vi "UHR-Fleezers Control (host) - 10.7.vi"() -> ()   [LabVIEW 2011] (continued)
        n1732 = Equal?(x=w2649, y=0) -> (x = y?=w2647:bool)
      }
      n1733 = local write "Stop All"(FALSE ("Stop All")) -> ()
    }
    frame #1 {
      n1734 = call "DMR_Init.vi"() -> ()  [unwired: 3 out]
    }
    frame #2 {
      # "Setting the destination format to Mono8 makes sure that the image can be displayed in the intensity plot."
      n1735 = call "DMR_GetDevice.vi"("search string IN"="DE019116701") -> ("device handle OUT"=w2672:i32)  [unwired: 4 in, 2 out]
      n1736 = call "DMR_OpenDevice.vi"("device handle IN"=w2672) -> ("driver handle OUT"=w2655:i32)  [unwired: 4 out]
      n1737 = call "DMR_FindList.vi"("flags IN"=u32 0 ("flags"), "list name IN"="" ("String"), "list type IN"=T31."camera descriptions", "driver handle IN"=w2655) -> ("list handle OUT"=w2658:i32)  [unwired: 2 out]
      n1738 = call "DMR_FindList.vi"("flags IN"=u32 0 ("flags"), "list name IN"="Base", "list type IN"=T31."setting", "driver handle IN"=w2655) -> ("list handle OUT"=w2656:i32)  [unwired: 2 out]
      n1739 = call "OBJ_GetHandle.vi"("object name IN"="VideoStandard", "list handle IN"=w2658) -> ("object handle OUT"=w2652:i32)  [unwired: 3 out]
      n1740 = call "OBJ_GetHandle.vi"("object name IN"="PixelFormat", "list handle IN"=w2656) -> ("object handle OUT"=w2666:i32)  [unwired: 3 out]
      n1741 = call "OBJ_SetS.vi"("value index IN"=0, "value IN"="NTSC M", "object handle IN"=w2652) -> ()  [unwired: 2 out]
      n1742 = call "OBJ_SetS.vi"("value index IN"=0, "value IN"="Mono8" ("value"), "object handle IN"=w2666) -> ()  [unwired: 2 out]
      n1743 = call "OBJ_GetHandle.vi"("object name IN"="VideoChannel", "list handle IN"=w2656) -> ("object handle OUT"=w2662:i32)  [unwired: 3 out]
      n1744 = while {
        tunnel: [w2677] -> w2654
        tunnel: w2655 -> [w2674]
        stop <- w2675 continue-if-true
        n1745 = call "DMR_ImageRequestSingle.vi"("request control IN"=0, "driver handle IN"=w2674) -> ("error code OUT"=w2676:i32, "driver handle OUT"=w2677:i32)  [unwired: 2 out]
        n1746 = Equal To 0?(x=w2676) -> (x = 0?=w2675:bool)
      }
      n1747 = call "OBJ_SetI.vi"("value index IN"=0, "value IN"=3 ("Video channel"), "object handle IN"=w2662) -> ()  [unwired: 2 out]
    }
    frame #3 {
      w2683 = T17 0 items=["Grayscale (U8)", "Grayscale (I16)", "Grayscale (SGL)", "Complex (CSG)", "RGB (U32)", "HSL (U32)", "RGB (U64)"] ("Image Type")
      w2691 = T17 0 items=["Grayscale (U8)", "Grayscale (I16)", "Grayscale (SGL)", "Complex (CSG)", "RGB (U32)", "HSL (U32)", "RGB (U64)"] ("Image Type")
      n1748 = for "Create Greyscale map" {
        N: 256 -> [_]
        tunnel: [w2697] -> w2680 mode=indexing
        workers-P: _ -> [_]
        i -> [w2700]
        n1749 = To Unsigned Byte Integer(number=w2700) -> (unsigned 8bit integer=w2696:u8)
        n1750 = Join Numbers(hi=w2696, lo=w2696) -> ((hi.lo)=w2699:u16)
        n1751 = Join Numbers(hi=w2696, lo=w2696) -> ((hi.lo)=w2698:u16)
        n1752 = Join Numbers(hi=w2699, lo=w2698) -> ((hi.lo)=w2697:u32)
      }
      n1753 = call "IMAQ Create"("Image Name"="Scaled video", "Image Type"=w2683) -> ("New Image"=w2682:T2)  [unwired: 2 in, 2 out]
      n1754 = call "IMAQ Create"("Image Name"="Main video", "Image Type"=w2691) -> ("New Image"=w2692:T2)  [unwired: 2 in, 2 out]
      n1755 = node-c288(0 ("Processor")) -> (w2690:T21)  [unwired: 3 out]
      n1756 = Initialize Array(u32 0 ("Window Number (0...15)"), 480 ("dimension size"), 640 ("dimension size")) -> (w2685:u32[][])
      n1757 = timed-loop {
        tunnel: w2695 -> [w2717]
        tunnel: [w2716] -> w2694
        tunnel: w2692 -> [w2715]
        timing: w2690 -> [_]
        timing-out: [_] -> w2689
        tunnel: w2685 -> [w2704]
        tunnel: w2682 -> [w2702]
        tunnel: w2680 -> [w2701]
        stop <- w2703 stop-if-true
        # "This block performs the \nactual image capture."
        n1758 = node-c288() -> ()  [unwired: 2 out]
        n1759 = local read "Stop All"() -> (w2703:bool)
        n1760 = Reciprocal(x="Video Capture Rate (Hz)") -> (1/x=w2707:dbl)
        n1761 = Multiply(x=w2707, y=1000.0) -> (x*y=w2705:dbl)
        n1762 = call "DMR_ImageRequestWaitFor.vi"("queue number IN"=0, "timeout(ms) IN"=500, "driver handle IN"=w2717) -> ("error code OUT"=w2721:i32, "request number OUT"=w2718:i32, "driver handle OUT"=w2719:i32)
        n1763 = feedback #1(T32 refnum ("Avi Refnum")) -> (w2709:T32)
        n1764 = case shown="True" "New Video File" {
          tunnel: [T32 refnum ("Avi Refnum") w2738] -> w2711
          tunnel: [FALSE TRUE] -> w2712
          tunnel: w2709 -> [_ w2734]
          frame False {
          }
          frame True {
            n1765 = call "Create new save file.vi"("Ext"=".avi" ("string"), "Index In"="Video Index") -> ("Path Out"=w2730:path, "Index Out"=w2731:dbl)  [unwired: 1 in]
            "Path Out" <- w2730
            n1766 = Not Equal?(x=w2734, y=T32 refnum ("Avi Refnum")) -> (x != y?=w2735:bool)
            n1767 = Increment(x=w2731) -> (x+1=w2740:dbl)
            n1768 = case shown="True" w2735 {
              tunnel: w2734 -> [_ w2741]
              frame False {
              }
              frame True {
                n1769 = call "IMAQ AVI Close"("Avi Refnum"=w2741) -> ()  [unwired: 1 in, 10 out]
              }
            }
            n1770 = local write "Video Index"(w2740) -> ()
            n1771 = call "IMAQ AVI Create"("Frames Per Second"=u32 30, "AVI Path"=w2730) -> ("Avi Refnum"=w2738:T32)  [unwired: 5 in, 4 out]
          }
        }
        n1772 = Equal To 0?(x=w2721) -> (x = 0?=w2720:bool)
        n1773 = Select(t=w2711, s=w2712, f=w2709) -> (s? t:f=w2710:T32)
        n1774 = feedback-in #1(w2710) -> ()
        n1775 = case shown="True" w2720 {
          tunnel: w2719 -> [w2742 w2767]
          tunnel: w2718 -> [_ w2766]
          tunnel: [w2742 w2763] -> w2716
          tunnel: w2715 -> [_ w2747]
          tunnel: w2704 -> [_ w2751]
          tunnel: w2710 -> [_ w2749]
          tunnel: w2702 -> [_ w2744]
          tunnel: w2701 -> [_ w2743]
          frame False {
          }
          frame True {
            w2757 = u32 0 ("X-offset IN")
            n1776 = call "DMR_GetImageRequestBufferData.vi"("driver handle IN"=w2767, "request number IN"=w2766) -> ("width OUT"=w2756:i32, "height OUT"=w2755:i32, "driver handle OUT"=w2762:i32, "request number OUT"=w2761:i32, "bytes per pixel OUT"=w2758:i32)  [unwired: 13 out]
            n1777 = call "DMR_GetImageRequestBufferImageData.vi"("driver handle IN"=w2762, "request number IN"=w2761, "bytes per pixel IN"=w2758, "X-offset IN"=w2757, "Y-offset IN"=w2757, "height IN"=w2755, "width IN"=w2756) -> ("driver handle OUT"=w2760:u32, "request number OUT"=w2759:u32, "image OUT"=w2752:u32[][])  [unwired: 10 out]
            n1778 = call "DMR_ImageRequestUnlock.vi"("request number IN"=w2759, "driver handle IN"=w2760) -> ("driver handle OUT"=w2765:i32)  [unwired: 1 in, 2 out]
            n1779 = case shown="True" "Averaging" {
              tunnel: w2752 -> [w2803 w2808]
              tunnel: [w2803 w2807] -> w2748
              tunnel: w2751 -> [_ w2805]
              frame False {
              }
              frame True {
                (unwired) 1
                w2813 = 1
                n1780 = feedback #2(w2805) -> (w2804:u32[][])
                n1781 = Add(x=w2808, y=w2804) -> (x+y=w2809:u32[][])
                n1782 = Select(t=w2805, s="Reset Averaging", f=w2809) -> (s? t:f=w2811:u32[][])
                n1783 = feedback-in #2(w2811) -> ()
                n1784 = feedback #3(w2813) -> (w2806:i32)
                n1785 = Divide(x=w2809, y=w2806) -> (x/y=w2810:dbl[][])
                n1786 = Increment(x=w2806) -> (x+1=w2814:i32)
                n1787 = To Unsigned Long Integer(number=w2810) -> (unsigned 32bit integer=w2807:u32[][])
                n1788 = Select(t=w2813, s="Reset Averaging", f=w2814) -> (s? t:f=w2812:i32)
                n1789 = feedback-in #3(w2812) -> ()
              }
            }
            n1790 = call "DMR_ImageRequestSingle.vi"("request control IN"=0, "driver handle IN"=w2765) -> ("driver handle OUT"=w2763:i32)  [unwired: 3 out]
            n1791 = disable-structure shown="Disabled" {
              disable-tunnel: w2748 -> [w2780 _]
              disable-tunnel: w2744 -> [w2779 _]
              frame Disabled {
                n1792 = To Double Precision Float(number=w2780) -> (double precision float=w2778:dbl[][])
                n1793 = In Range and Coerce(upper limit="Intensity Upper", x=w2778, lower limit="Intensity Lower") -> (coerced(x)=w2777:dbl[][])  [unwired: 1 out]
                n1794 = Subtract(x="Intensity Upper", y="Intensity Lower") -> (x-y=w2774:dbl)
                n1795 = Subtract(x=w2777, y="Intensity Lower") -> (x-y=w2775:dbl[][])
                n1796 = Divide(x=w2775, y=w2774) -> (x/y=w2776:dbl[][])
                n1797 = Multiply(x=255.0, y=w2776) -> (x*y=w2772:dbl[][])
                n1798 = To Unsigned Byte Integer(number=w2772) -> (unsigned 8bit integer=w2781:u8[][])
                n1799 = call "IMAQ ArrayToImage"("Image Pixels (U8)"=w2781, "Image"=w2779) -> ("Image Out"=w2768:T2)  [unwired: 4 in, 5 out]
                n1800 = First Call?() -> (First Call?: T/F=w2769:bool)
                n1801 = case shown="True" w2769 {
                  tunnel: w2768 -> [w2782 w2793]
                  frame False {
                    n1802 = flat-sequence {
                      tunnel: w2782 -> [w2788]
                      frame #0 {
                        w2785 = FALSE ("Get/Set Status? (Set)")
                        w2784 = 0 ("Window Number (0...15)")
                        n1803 = call "IMAQ WindSize"("Get/Set Status? (Set)"=w2785, "Window Number"=w2784) -> ("Width & Height out"=→"Window Size":cluster{"Width":i32, "Height":i32})  [unwired: 4 in, 2 out]
                        n1804 = call "IMAQ WindMove"("Window Number (0...15)"=w2784, "Get/Set Status? (Set)"=w2785) -> ("Coordinates (screen)"=→"Window Position":cluster{"X Position":i32, "Y Position":i32})  [unwired: 3 in, 1 out]
                        n1805 = call "IMAQ WindDraw"("Resize to Image Size? (Y)"=FALSE, "Window Number (0...15)"=w2784, "Image"=w2788) -> ()  [unwired: 7 in, 2 out]
                      }
                      frame #1 {
                        n1806 = call "IMAQ WindZoom 2"("Center Point"="Center Point", "Zoom to Fit? (False)"=FALSE, "Zoom Factor"="Zoom Factor") -> ()  [unwired: 5 in, 4 out]
                      }
                    }
                  }
                  frame True {
                    n1807 = flat-sequence {
                      tunnel: w2793 -> [w2796]
                      tunnel: [w2794] -> w2792
                      tunnel: w2792 -> [w2798]
                      frame #0 {
                        w2795 = TRUE ("Resize to Image Size? (Y)")
                        w2794 = 0 ("Window Number (0...15)")
                        n1808 = call "IMAQ WindNonTearing"("Window Number"=w2794, "NonTearing? (True)"=w2795) -> ()  [unwired: 8 in, 2 out]
                        n1809 = call "IMAQ WindDraw"("Resize to Image Size? (Y)"=w2795, "Window Number (0...15)"=w2794, "Image"=w2796) -> ()  [unwired: 7 in, 2 out]
                      }
                      frame #1 {
                        n1810 = call "IMAQ WindSize"("Scrollbars? (N)"=FALSE, "Width & Height"="Initial Window Size", "Window Number"=w2798) -> ()  [unwired: 3 in, 3 out]
                        n1811 = call "IMAQ WindMove"("Window Number (0...15)"=w2798, "Coordinates (screen)"="Initial Window Position") -> ()  [unwired: 3 in, 2 out]
                      }
                    }
                  }
                }
              }
              frame Enabled {
              }
            }
            n1812 = To Unsigned Byte Integer(number=w2748) -> (unsigned 8bit integer=w2746:u8[][])
            n1813 = call "IMAQ ArrayToImage"("Image Pixels (U8)"=w2746, "Image"=w2747) -> ("Image Out"=w2745:T2)  [unwired: 4 in, 5 out]
            "Primary Video Display" <- w2745
            n1814 = case shown="True" "Save Video" {
              tunnel: w2749 -> [_ w2802]
              tunnel: w2745 -> [_ w2801]
              frame False {
              }
              frame True {
                n1815 = call "IMAQ AVI Write Frame"("Image"=w2801, "Avi Refnum"=w2802) -> ()  [unwired: 2 in, 8 out]
              }
            }
            n1816 = case shown="True" "Save Image" {
              tunnel: w2746 -> [_ w2817]
              tunnel: w2743 -> [_ w2816]
              frame False {
              }
              frame True {
                n1817 = call <vilib>:"Flatten Pixmap.vi"("colors"=w2816, "8-bit pixmap"=w2817) -> ("image data"=w2823:T33)  [unwired: 4 in, 5 out]
                n1818 = call "Create new save file.vi"("Insert"="video_frame_" ("string"), "Ext"=".bmp" ("string"), "Index In"="Image Index") -> ("Path Out"=w2819:path, "Index Out"=w2824:dbl)
                n1819 = Increment(x=w2824) -> (x+1=w2818:dbl)
                n1820 = local write "Image Index"(w2818) -> ()
                n1821 = call <vilib>:"Write BMP File.vi"("image data"=w2823, "path to BMP file"=w2819) -> ()  [unwired: 1 in, 9 out]
              }
            }
          }
        }
        n1822 = node-c288(w2705) -> ()  [unwired: 1 out]
      }
      n1823 = node-c288(w2689) -> ()  [unwired: 1 out]
      n1824 = call "DMR_CloseDevice.vi"("driver handle IN"=w2694) -> ()  [unwired: 1 in, 4 out]
    }
    frame #4 {
      n1825 = call "DMR_Close.vi"() -> ()  [unwired: 1 out]
    }
  }
  n1826 = node-c288(i64 1 ("Period"), 1 ("Processor")) -> (w175:T21)  [unwired: 2 out]
  n1827 = timed-loop "Acquire Data" {
    tunnel: w50 -> [w3123]
    tunnel: w49 -> [w3122]
    tunnel: [w3152] -> w270
    tunnel: [w3147] -> w268
    timing: w175 -> [_]
    timing-out: [_] -> w174
    tunnel: w69 -> [w2960]
    stop <- "Stop All" stop-if-true
    w2875 = "Initialize"
    w2945 = "NI_ChannelName" ("name")
    n1828 = node-c288() -> ()  [unwired: 2 out]
    n1829 = First Call?() -> (First Call?: T/F=w2910:bool)
    n1830 = Or(x="Reset", y=w2910) -> (x .or. y?=w2911:bool)
    n1831 = local read "Flushing P1"() -> (w2829:bool)
    n1832 = case "Reset data stream" shown="True" w2911 {
      tunnel: w3123 -> [w4128 w4136]
      tunnel: w3122 -> [w4127 w4135]
      tunnel: [w4128 w4130] -> w3118
      tunnel: [w4127 w4129] -> w3117
      frame False {
      }
      frame True {
        w4133 = TRUE ("AI to FIFO")
        n1833 = local write "Overflow (data lost)"(FALSE ("Overflow (data lost)")) -> ()
        n1834 = call "reset FPGA DMA.vi"("error in"=w4135, "FPGA VI Reference In"=w4136) -> ("error out"=w4131:errorcluster, "FPGA VI Reference Out"=w4132:T19)
        n1835 = xnode "Read/Write Control"("FPGA VI Reference In"=w4132, "error in"=w4131, "AI to FIFO"=w4133, "APD to FIFO"=w4133) -> ("FPGA VI Reference Out"=w4130:T19, "error out"=w4129:errorcluster)
      }
    }
    n1836 = case shown="True" w2829 {
      frame False {
      }
      frame True {
        n1837 = local read "Flush rate (uL/m) P1"() -> (w3169:dbl)
        n1838 = local read "HP1 Flush Time (s)"() -> (w3178:dbl)
        n1839 = local read "DMA Update Period (s)"() -> (w3172:dbl)
        n1840 = Divide(x=w3169, y=60.0) -> (x/y=w3170:dbl)
        n1841 = Divide(x=w3178, y=w3172) -> (x/y=w3167:dbl)
        n1842 = feedback #4(0) -> (w3176:i32)
        n1843 = Increment(x=w3176) -> (x+1=w3166:i32)
        n1844 = Greater?(x=w3166, y=w3167) -> (0:w3175:bool)
        n1845 = Compound Arithmetic op=MULTIPLY(w3172, w3166, w3170) -> (→"P1 Flush Volume (uL)":dbl)
        n1846 = Divide(x=w3166, y=w3167) -> (x/y=→"P1 Flushing Bar":dbl)
        n1847 = case shown="True" w3175 {
          tunnel: w3166 -> [w3179 _]
          tunnel: [w3179 0] -> w3174
          frame False {
          }
          frame True {
            w3180 = FALSE ("Flushing P1")
            n1848 = local write "Inject Pump 1"(w3180) -> ()
            n1849 = local write "Flushing P1"(w3180) -> ()
            n1850 = property on="Clear Volume P1" class="Bool (strict)"("Val(Sgnl)"=TRUE ("Value (Signaling)")) -> ()  [unwired: 2 in, 2 out]
          }
        }
        n1851 = feedback-in #4(w3174) -> ()
      }
    }
    n1852 = Or(x="Start AOD Scan", y="Trap Raster Scan") -> (x .or. y?=w3068:bool)
    n1853 = case "Start AOM raster scan" shown="True" w3068 {
      tunnel: w3118 -> [w3978 w3988]
      tunnel: w3117 -> [w3977 w3987]
      tunnel: [w3978 w3981] -> w3116
      tunnel: [w3977 w3980] -> w3115
      frame False {
      }
      frame True {
        n1854 = case shown="True" "Restart DMA? (AOD)" {
          tunnel: [w4026 w4028] -> w3982
          tunnel: [w4025 w4027] -> w3983
          tunnel: w3988 -> [w4026 w4030]
          tunnel: w3987 -> [w4025 w4029]
          frame False {
          }
          frame True {
            n1855 = local write "Overflow (data lost)"(FALSE ("Overflow (data lost)")) -> ()
            n1856 = call "reset FPGA DMA.vi"("error in"=w4029, "FPGA VI Reference In"=w4030) -> ("error out"=w4027:errorcluster, "FPGA VI Reference Out"=w4028:T19)
          }
        }
        n1857 = local write "Trap Raster Scan"(FALSE ("Trap Raster Scan")) -> ()
        n1858 = case shown="True" "Move MCL Also?" {
          tunnel: w3983 -> [w3991 w4020]
          tunnel: w3982 -> [w3992 w4021]
          tunnel: [w3990 w4024] -> w3981
          tunnel: [w3989 w4023] -> w3980
          frame False {
            w3993 = TRUE ("AI to FIFO")
            n1859 = xnode "Read/Write Control"("FPGA VI Reference In"=w3992, "error in"=w3991, "AI to FIFO"=w3993, "APD to FIFO"=w3993, "Start scan"=w3993) -> ("FPGA VI Reference Out"=w3990:T19, "error out"=w3989:errorcluster)
          }
          frame True {
            w4017 = FALSE ("1D or 2D Scan?")
            w4022 = TRUE ("AI to FIFO")
            # "Count for MCL loop"
            # "N total cycles"
            # "N steps"
            # "V_int"
            n1860 = local read "Scan Range (nm)"() -> (w3999:dbl)
            n1861 = local read "Number of F/B Scans (AOD)"() -> (w4016:u16)
            n1862 = Sign(1:w3999) -> (0:w3998:dbl)
            n1863 = Compound Arithmetic op=MULTIPLY(w3999, "MCL Step Position Ratio", "MCL/AOM Scale Tweak") -> (w4003:dbl)
            n1864 = Negate(x=w3998) -> (-x=w3995:dbl)
            n1865 = Multiply(x=w3995, y="MCL Step Increment (V_int)") -> (x*y=w3997:dbl)
            n1866 = Divide(x=w4003, y="MCL X Cal (nm/V)") -> (x/y=w4009:dbl)
            n1867 = Multiply(x=32767.0 ("y"), y=w4009) -> (x*y=w4015:dbl)
            n1868 = local read "Total Counts (ticks)"() -> (w4000:u32)
            n1869 = local read "Cycles/step (AOD)"() -> (w4011:u64)
            n1870 = local read "Scan steps (AOD)"() -> (w4012:u64)
            n1871 = Divide(x=w4015, y=10.0) -> (x/y=w4008:dbl)
            n1872 = Divide(x=w4008, y="MCL Step Increment (V_int)") -> (x/y=w4006:dbl)
            n1873 = Absolute Value(x=w4006) -> (abs(x)=w3994:dbl)
            n1874 = Compound Arithmetic op=MULTIPLY(w4012, w4011, w4000) -> (w4007:u64)
            n1875 = local write "wait to reset values"(w4022) -> ()
            n1876 = local write "MCL Scanning"(w4022) -> ()
            n1877 = Divide(x=w4007, y=w3994) -> (x/y=w4004:dbl)
            "MCL Count" <- w4004
            n1878 = xnode "Read/Write Control"("FPGA VI Reference In"=w4021, "error in"=w4020, "Scan steps (MCL)"=w3994, "Number of scans (MCL)"=w4016, "Cycles per step (MCL)"=u64 1, "Scan freq.  increment (MCL)"=w3997, "1D or 2D Scan?"=w4017, "MCL Scan Axis"=w4017, "Cont. Scan (MCL)"=w4017, "MCL count"=w4004) -> ("FPGA VI Reference Out"=w4019:T19, "error out"=w4018:errorcluster)
            n1879 = xnode "Read/Write Control"("FPGA VI Reference In"=w4019, "error in"=w4018, "AI to FIFO"=w4022, "APD to FIFO"=w4022, "Start scan"=w4022, "Start scan (MCL)"=w4022) -> ("FPGA VI Reference Out"=w4024:T19, "error out"=w4023:errorcluster)
          }
        }
        "Raster Scanning..." <- TRUE ("Scanning...")
      }
    }
    n1880 = local read "Flushing P3"() -> (w2830:bool)
    n1881 = case "Keep track of when Harvard Pump 3 is done flushing" shown="True" w2830 {
      frame False {
      }
      frame True {
        n1882 = local read "Flush rate (uL/m) P3"() -> (w3186:dbl)
        n1883 = local read "DMA Update Period (s)"() -> (w3188:dbl)
        n1884 = local read "HP3 Flush Time (s)"() -> (w3195:dbl)
        n1885 = Divide(x=w3186, y=60.0) -> (x/y=w3184:dbl)
        n1886 = feedback #5(0) -> (w3193:i32)
        n1887 = Increment(x=w3193) -> (x+1=w3187:i32)
        n1888 = Divide(x=w3195, y=w3188) -> (x/y=w3189:dbl)
        n1889 = Greater?(x=w3187, y=w3189) -> (0:w3192:bool)
        n1890 = Compound Arithmetic op=MULTIPLY(w3188, w3187, w3184) -> (→"P3 Flush Volume (uL)":dbl)
        n1891 = case shown="True" w3192 {
          tunnel: w3187 -> [w3196 _]
          tunnel: [w3196 0] -> w3191
          frame False {
          }
          frame True {
            w3197 = FALSE ("Flushing P3")
            n1892 = local write "Inject Pump 3"(w3197) -> ()
            n1893 = local write "Flushing P3"(w3197) -> ()
            n1894 = property on="Clear Volume P3" class="Bool (strict)"("Val(Sgnl)"=TRUE ("Value (Signaling)")) -> ()  [unwired: 2 in, 2 out]
          }
        }
        n1895 = feedback-in #5(w3191) -> ()
        n1896 = Divide(x=w3187, y=w3189) -> (x/y=→"P3 Flushing Bar":dbl)
      }
    }
    n1897 = And(x="Save scans", y=w3068) -> (x .and. y?=w3114:bool)
    n1898 = Compound Arithmetic op=OR("Start MCL Scan", "Confocal Image", "Confocal Linescan") -> (w3066:bool)
    n1899 = And(x="Save Data (MCL)", y=w3066) -> (x .and. y?=w3113:bool)
    n1900 = case "Start MCL raster scan" shown="True" w3066 {
      tunnel: w3116 -> [w3595 w3611]
      tunnel: w3115 -> [w3594 w3610]
      tunnel: [w3595 w3606] -> w2958
      tunnel: [w3594 w3605] -> w2957
      tunnel: [FALSE w3604] -> w3099
      tunnel: "Start MCL Scan" -> [_ w3599]
      tunnel: "Confocal Image" -> [_ w3598]
      tunnel: "Confocal Linescan" -> [_ _]
      frame False {
      }
      frame True {
        w3604 = TRUE
        n1901 = case shown="True" "Restart DMA? (MCL)" {
          tunnel: [w3656 w3658] -> w3609
          tunnel: [w3655 w3657] -> w3608
          tunnel: w3611 -> [w3656 w3661]
          tunnel: w3610 -> [w3655 w3660]
          frame False {
          }
          frame True {
            n1902 = call "reset FPGA DMA.vi"("error in"=w3660, "FPGA VI Reference In"=w3661) -> ("error out"=w3657:errorcluster, "FPGA VI Reference Out"=w3658:T19)
            n1903 = local write "Overflow (data lost)"(FALSE ("Overflow (data lost)")) -> ()
          }
        }
        n1904 = case shown="False" w3599 {
          selector: w3599 -> [_ w3615]
          tunnel: w3598 -> [w3614 _]
          tunnel: [w3614 w3615] -> w3597
          frame False {
            n1905 = property on="2D or 1D Scan" class="Bool (strict)"("Val(Sgnl)"=w3614) -> ()  [unwired: 2 in, 2 out]
            n1906 = property on="Confocal Image" class="Bool (strict)"("Value"=FALSE ("Start Confocal Map")) -> ()  [unwired: 2 in, 2 out]
          }
          frame True {
          }
        }
        n1907 = local write "MCL Scanning"(w3604) -> ()
        n1908 = local read "AO1"() -> (w3601:dbl)
        n1909 = local read "AO2"() -> (w3600:dbl)
        n1910 = case shown="True" "Center Scan" {
          tunnel: w3609 -> [w3622 w3654]
          tunnel: w3608 -> [w3621 w3653]
          tunnel: [w3620 w3652] -> w3606
          tunnel: [w3619 w3651] -> w3605
          tunnel: [w3617 w3638] -> w3603
          tunnel: [w3616 w3637] -> w3602
          tunnel: w3601 -> [w3617 w3643]
          tunnel: w3600 -> [w3616 w3646]
          tunnel: w3597 -> [_ _]
          frame False {
            w3618 = TRUE ("AI to FIFO")
            n1911 = xnode "Read/Write Control"("FPGA VI Reference In"=w3622, "error in"=w3621, "AI to FIFO"=w3618, "APD to FIFO"=w3618, "Start scan (MCL)"=w3618) -> ("FPGA VI Reference Out"=w3620:T19, "error out"=w3619:errorcluster)
          }
          frame True {
            w3650 = TRUE ("AI to FIFO")
            n1912 = local read "Scan steps (MCL)"() -> (w3629:u64)
            n1913 = local read "Scan lines (y)"() -> (w3625:u64)
            n1914 = local read "Fast Scan Dir"() -> (w3636:bool)
            n1915 = local read "Actual MCL Inc (V)"() -> (w3626:dbl)
            n1916 = Decrement(x=w3625) -> (x-1=w3624:u64)
            n1917 = Decrement(x=w3629) -> (x-1=w3628:u64)
            n1918 = Multiply(x=w3626, y=w3624) -> (x*y=w3623:dbl)
            n1919 = Divide(x=w3623, y=2.0) -> (x/y=w3633:dbl)
            n1920 = Multiply(x=w3626, y=w3628) -> (x*y=w3627:dbl)
            n1921 = Divide(x=w3627, y=2.0) -> (x/y=w3632:dbl)
            n1922 = Select(t=w3632, s=w3636, f=w3633) -> (s? t:f=w3631:dbl)
            n1923 = Select(t=w3633, s=w3636, f=w3632) -> (s? t:f=w3635:dbl)
            n1924 = Subtract(x=w3643, y=w3635) -> (x-y=w3634:dbl)
            n1925 = Subtract(x=w3646, y=w3631) -> (x-y=w3630:dbl)
            n1926 = local read "2D or 1D Scan"() -> (w3648:bool)
            n1927 = Not(x=w3636) -> (.not. x?=w3642:bool)
            n1928 = Not(x=w3648) -> (.not. x?=w3644:bool)
            n1929 = And(x=w3636, y=w3644) -> (x .and. y?=w3645:bool)
            n1930 = And(x=w3644, y=w3642) -> (x .and. y?=w3647:bool)
            n1931 = Select(t=w3646, s=w3647, f=w3630) -> (s? t:f=w3637:dbl)
            n1932 = Select(t=w3643, s=w3645, f=w3634) -> (s? t:f=w3638:dbl)
            n1933 = call "Volt to I16.vi"("Voltage In"=w3638) -> ("I16 Voltage Out"=w3641:i16)
            n1934 = call "Volt to I16.vi"("Voltage In"=w3637) -> ("I16 Voltage Out"=w3640:i16)
            n1935 = xnode "Read/Write Control"("FPGA VI Reference In"=w3654, "error in"=w3653, "AI to FIFO"=w3650, "APD to FIFO"=w3650, "Start scan (MCL)"=w3650, "AO1"=w3641, "AO2"=w3640) -> ("FPGA VI Reference Out"=w3652:T19, "error out"=w3651:errorcluster)
          }
        }
        "Initial Y" <- w3603
        "Initial X" <- w3602
        n1936 = local write "Tab Control 6"(T3."Imaging" ("Tab Control 6")) -> ()
        "wait to reset values" <- w3604
      }
    }
    n1937 = local read "Trap Pos Elements/DMA read"() -> (w2954:u32)
    n1938 = local read "Trap AI Elements/DMA read"() -> (w3029:u32)
    n1939 = local read "APD Elements/DMA read"() -> (w2995:u32)
    n1940 = xnode "Get APD Data"("FPGA VI Reference In"=w2958, "error in"=w2957, "Number of Elements"=w2995, "Timeout (ms)"=-1) -> ("Data"=w2994:u32[], "Elements Remaining"=→"APD FIFO Elements Remaining":u32)  [unwired: 2 out]
    n1941 = xnode "Invoke Method"("FPGA VI Reference In"=w2958, "error in"=w2957, "Number of Elements"=w2954, "Timeout (ms)"=-1) -> ("Data"=w2917:u16[], "Elements Remaining"=→"Trap Pos FIFO El Remaining":u32)  [unwired: 2 out]
    n1942 = xnode "Get Trap Data"("FPGA VI Reference In"=w2958, "error in"=w2957, "Number of Elements"=w3029, "Timeout (ms)"=-1 ("Timeout")) -> ("FPGA VI Reference Out"=w2851:T19, "error out"=w2850:errorcluster, "Data"=w2918:i16[], "Elements Remaining"=w3160:u32)
    "FIFO El. Rem." <- w3160
    n1943 = local read "Trap AI FIFO Depth"() -> (w3162:u32)
    n1944 = Subtract(x=w3162, y=w3029) -> (x-y=w3161:u32)
    n1945 = Decimate 1D Array(w2917) -> (w2914:u16[], w2916:u16[], w2915:u16[])
    n1946 = Divide(x=w3160, y=w3161) -> (x/y=w3159:dbl)
    "Buffer Status" <- w3159
    n1947 = To Unsigned Long Integer(number=w2914) -> (unsigned 32bit integer=w2913:u32[])
    n1948 = Join Numbers(hi=w2916, lo=w2915) -> ((hi.lo)=w2912:u32[])
    n1949 = Equal?(x=w3159, y=1.0) -> (x = y?=w3157:bool)
    n1950 = Join Numbers(hi=w2913, lo=w2912) -> ((hi.lo)=w2906:u64[])
    n1951 = call "IR AOM word to freq - vec.vi"("Frequency Word In (double vec)"=w2906) -> ("Frequency Out"=w2953:dbl[])
    n1952 = case "Alert buffer overflow" shown="True" w3157 {
      frame False {
      }
      frame True {
        n1953 = call <vilib>:"Beep.vi"() -> ()  [unwired: 3 in, 9 out]
        "Overflow (data lost)" <- TRUE ("Overflow (data lost)")
      }
    }
    n1954 = Decimate 1D Array(w2953) -> (w2952:dbl[], w2951:dbl[])
    n1955 = Build Array(w2952, w2951) -> (w2950:dbl[][])
    n1956 = local read "Trap Sets"() -> (w3028:u32)
    n1957 = case "Deinterlace trap data, average down PSD" shown="2" w3028 {
      tunnel: w2918 -> [w3691 w3756]
      tunnel: [w3688 w3753] -> w3021
      tunnel: [w3691 w3755] -> w2909
      tunnel: "Detector Type" -> [w3690 w3751]
      tunnel: [w3689 w3754] -> w3020
      tunnel: [w3687 w3752] -> w3134
      frame 1, Default {
        n1958 = Divide(x=w3691, y=3276.7) -> (x/y=w3692:dbl[])
        n1959 = Decimate 1D Array(w3692) -> (w3701:dbl[], w3700:dbl[], w3699:dbl[], w3698:dbl[], w3697:dbl[], w3696:dbl[], w3695:dbl[], w3694:dbl[])
        n1960 = case shown="\"IR-QPD + PSD + FB-QPD position\"" w3690 {
          tunnel: w3701 -> [w3725 w3750]
          tunnel: w3700 -> [w3724 w3749]
          tunnel: w3699 -> [w3709 w3727]
          tunnel: w3698 -> [w3710 w3737]
          tunnel: w3697 -> [w3723 w3748]
          tunnel: w3696 -> [w3722 w3747]
          tunnel: w3695 -> [w3706 w3728]
          tunnel: w3694 -> [w3705 w3726]
          tunnel: [w3704 w3734] -> w3689
          tunnel: [w3703 w3733] -> w3688
          tunnel: [w3702 w3732] -> w3687
          frame "IR-QPD + PSD + FB-QPD", Default {
            w3702 = 0  # Channel pattern
            n1961 = Divide(x=w3725, y=w3710) -> (x/y=w3712:dbl[])
            n1962 = Divide(x=w3724, y=w3710) -> (x/y=w3711:dbl[])
            n1963 = Divide(x=w3723, y=w3706) -> (x/y=w3708:dbl[])
            n1964 = Divide(x=w3722, y=w3705) -> (x/y=w3707:dbl[])
            n1965 = Build Array(w3712, w3711, w3710, w3709, w3708, w3707, w3706, w3705) -> (w3703:dbl[][])
            n1966 = Bundle("T1 Y", "T1 X", "T1 Sum", "FB Sum", "PSD Y", "PSD X", "PSD Y Sum", "PSD X Sum") -> (w3721:T40)  [unwired: 1 out]
            n1967 = Cluster To Array(cluster=w3721) -> (array=w3704:string[])
          }
          frame "IR-QPD + PSD + FB-QPD position" {
            w3732 = 3  # Channel pattern
            n1968 = Negate(x=w3728) -> (-x=w3729:dbl[])
            n1969 = Divide(x=w3750, y=w3737) -> (x/y=w3739:dbl[])
            n1970 = Divide(x=w3749, y=w3737) -> (x/y=w3738:dbl[])
            n1971 = Divide(x=w3748, y=w3728) -> (x/y=w3736:dbl[])
            n1972 = Divide(x=w3747, y=w3729) -> (x/y=w3735:dbl[])
            n1973 = Build Array(w3739, w3738, w3737, w3726, w3727, w3736, w3735, w3728) -> (w3733:dbl[][])
            n1974 = Bundle("T1 Y", "T1 X", "T1 Sum", "FB X", "FB Sum", "PSD Y", "PSD X", "PSD Y Sum") -> (w3746:T40)  [unwired: 1 out]
            n1975 = Cluster To Array(cluster=w3746) -> (array=w3734:string[])
          }
        }
      }
      frame 2 {
        n1976 = case shown="\"IR-QPD + PSD + FB-QPD X position\"" w3751 {
          tunnel: w3756 -> [w3818 w3885 w3956]
          tunnel: [w3757 w3876 w3887] -> w3755
          tunnel: [w3784 w3867 w3934] -> w3754
          tunnel: [w3783 w3830 w3901] -> w3753
          tunnel: [w3777 w3865 w3932] -> w3752
          frame "IR-QPD + PSD + FB-QPD", Default {
            w3777 = 1  # Channel pattern
            # "time average x2 the 4th signal and the 4 psd signals (detection laser)"
            # "deinterlace 3 signals from qpd"
            n1977 = Decimate 1D Array(w3818) -> (w3817:i16[], w3816:i16[], w3782:i16[], w3815:i16[], w3805:i16[], w3803:i16[], w3802:i16[], w3800:i16[])
            n1978 = Decimate 1D Array(w3782) -> (w3781:i16[], w3780:i16[])
            n1979 = Decimate 1D Array(w3817) -> (w3814:i16[], w3786:i16[])
            n1980 = Decimate 1D Array(w3816) -> (w3813:i16[], w3811:i16[])
            n1981 = Decimate 1D Array(w3815) -> (w3812:i16[], w3810:i16[])
            n1982 = call "downsample 1D array - double.vi"("Ave N"=2.0, "Array In"=w3805) -> ("Array Out"=w3804:dbl[])  [unwired: 1 out]
            n1983 = call "downsample 1D array - double.vi"("Ave N"=2.0, "Array In"=w3803) -> ("Array Out"=w3785:dbl[])  [unwired: 1 out]
            n1984 = call "downsample 1D array - double.vi"("Ave N"=2.0, "Array In"=w3802) -> ("Array Out"=w3801:dbl[])  [unwired: 1 out]
            n1985 = call "downsample 1D array - double.vi"("Ave N"=2.0, "Array In"=w3800) -> ("Array Out"=w3799:dbl[])  [unwired: 1 out]
            n1986 = Interleave 1D Arrays(w3814, w3813, w3812, w3786, w3811, w3810, w3781, w3780, w3804, w3785, w3801, w3799) -> (w3798:dbl[])
            n1987 = Divide(x=w3798, y=3276.7) -> (x/y=w3797:dbl[])
            n1988 = Decimate 1D Array(w3797) -> (w3796:dbl[], w3795:dbl[], w3794:dbl[], w3793:dbl[], w3792:dbl[], w3791:dbl[], w3779:dbl[], w3778:dbl[], w3790:dbl[], w3789:dbl[], w3788:dbl[], w3787:dbl[])
            n1989 = Divide(x=w3796, y=w3794) -> (x/y=w3764:dbl[])
            n1990 = Divide(x=w3795, y=w3794) -> (x/y=w3763:dbl[])
            n1991 = Divide(x=w3793, y=w3791) -> (x/y=w3762:dbl[])
            n1992 = Divide(x=w3792, y=w3791) -> (x/y=w3761:dbl[])
            n1993 = Divide(x=w3790, y=w3788) -> (x/y=w3760:dbl[])
            n1994 = Divide(x=w3789, y=w3787) -> (x/y=w3759:dbl[])
            n1995 = Build Array(w3764, w3763, w3794, w3762, w3761, w3791, w3779, w3778, w3760, w3759, w3788, w3787) -> (w3783:dbl[][])
            n1996 = Bundle("T1 Y", "T1 X", "T1 Sum", "T2 Y", "T2 X", "T2 Sum", "T1 FB Sum", "T2 FB Sum", "PSD Y", "PSD X", "PSD Y Sum", "PSD X Sum") -> (w3765:T41)  [unwired: 1 out]
            n1997 = To Word Integer(number=w3798) -> (16bit integer=w3757:i16[])
            n1998 = Cluster To Array(cluster=w3765) -> (array=w3784:string[])
          }
          frame "IR-QPD + PSD + FB-QPD X position" {
            w3865 = 2  # Channel pattern
            # "time average x2 the 3 psd signals (detection laser)"
            # "deinterlace 3 signals from qpds"
            n1999 = Decimate 1D Array(w3885) -> (w3884:i16[], w3883:i16[], w3866:i16[], w3882:i16[], w3828:i16[], w3825:i16[], w3822:i16[], w3853:i16[])
            n2000 = Decimate 1D Array(w3866) -> (w3851:i16[], w3849:i16[])
            n2001 = Decimate 1D Array(w3884) -> (w3881:i16[], w3868:i16[])
            n2002 = Decimate 1D Array(w3883) -> (w3880:i16[], w3878:i16[])
            n2003 = Decimate 1D Array(w3882) -> (w3879:i16[], w3877:i16[])
            n2004 = Decimate 1D Array(w3853) -> (w3852:i16[], w3850:i16[])
            n2005 = call "downsample 1D array - I16.vi"("Ave N"=2.0, "Array In"=w3828) -> ("Array Out"=w3826:i16[])  [unwired: 1 in]
            n2006 = call "downsample 1D array - I16.vi"("Ave N"=2.0, "Array In"=w3822) -> ("Array Out"=w3820:i16[])  [unwired: 1 in]
            n2007 = call "downsample 1D array - I16.vi"("Ave N"=2.0, "Array In"=w3825) -> ("Array Out"=w3823:i16[])  [unwired: 1 in]
            n2008 = Interleave 1D Arrays(w3881, w3880, w3879, w3868, w3878, w3877, w3852, w3851, w3850, w3849, w3826, w3823, w3820) -> (w3876:i16[])
            n2009 = Divide(x=w3876, y=3276.7) -> (x/y=w3875:dbl[])
            n2010 = Decimate 1D Array(w3875) -> (w3874:dbl[], w3873:dbl[], w3872:dbl[], w3871:dbl[], w3870:dbl[], w3869:dbl[], w3841:dbl[], w3839:dbl[], w3838:dbl[], w3836:dbl[], w3835:dbl[], w3834:dbl[], w3831:dbl[])
            n2011 = Negate(x=w3831) -> (-x=w3829:dbl[])
            n2012 = Divide(x=w3835, y=w3831) -> (x/y=w3833:dbl[])
            n2013 = Divide(x=w3834, y=w3829) -> (x/y=w3832:dbl[])
            n2014 = Divide(x=w3874, y=w3872) -> (x/y=w3857:dbl[])
            n2015 = Divide(x=w3873, y=w3872) -> (x/y=w3856:dbl[])
            n2016 = Divide(x=w3871, y=w3869) -> (x/y=w3855:dbl[])
            n2017 = Divide(x=w3870, y=w3869) -> (x/y=w3854:dbl[])
            n2018 = Divide(x=w3841, y=w3839) -> (x/y=w3840:dbl[])
            n2019 = Divide(x=w3838, y=w3836) -> (x/y=w3837:dbl[])
            n2020 = Build Array(w3857, w3856, w3872, w3855, w3854, w3869, w3840, w3839, w3837, w3836, w3833, w3832, w3831) -> (w3830:dbl[][])
            n2021 = Bundle("T1 Y", "T1 X", "T1 Sum", "T2 Y", "T2 X", "T2 Sum", "T1 FB X", "T1 FB Sum", "T2 FB X", "T2 FB Sum", "PSD Y", "PSD X", "PSD Y Sum") -> (w3858:T42)  [unwired: 1 out]
            n2022 = Cluster To Array(cluster=w3858) -> (array=w3867:string[])
          }
          frame "IR-QPD + PSD + FB-QPD XY positions" {
            w3932 = 4  # Channel pattern
            # "time average x2 the 3 psd signals (detection laser)"
            # "deinterlace 3 signals from qpds"
            n2023 = Decimate 1D Array(w3956) -> (w3955:i16[], w3954:i16[], w3933:i16[], w3953:i16[], w3899:i16[], w3945:i16[], w3944:i16[], w3921:i16[])
            n2024 = Decimate 1D Array "Feedback Sum"(w3933) -> (w3917:i16[], w3915:i16[])
            n2025 = Decimate 1D Array "QPD Y"(w3955) -> (w3952:i16[], w3935:i16[])
            n2026 = Decimate 1D Array "QPD X"(w3954) -> (w3951:i16[], w3949:i16[])
            n2027 = Decimate 1D Array "Feedback Y"(w3899) -> (w3898:i16[], w3897:i16[])
            n2028 = Decimate 1D Array "QPD Sum"(w3953) -> (w3950:i16[], w3948:i16[])
            n2029 = Decimate 1D Array "Feedback X"(w3921) -> (w3918:i16[], w3916:i16[])
            n2030 = call "downsample 1D array - double.vi"("Ave N"=2.0, "Array In"=w3945) -> ("Array Out"=w3920:dbl[])  [unwired: 1 out]
            n2031 = call "downsample 1D array - double.vi"("Ave N"=2.0, "Array In"=w3944) -> ("Array Out"=w3919:dbl[])  [unwired: 1 out]
            n2032 = Interleave 1D Arrays(w3952, w3951, w3950, w3935, w3949, w3948, w3898, w3918, w3917, w3897, w3916, w3915, w3920, w3919) -> (w3943:dbl[])
            n2033 = Divide(x=w3943, y=3276.7) -> (x/y=w3942:dbl[])
            n2034 = Decimate 1D Array(w3942) -> (w3941:dbl[], w3940:dbl[], w3939:dbl[], w3938:dbl[], w3937:dbl[], w3936:dbl[], w3894:dbl[], w3908:dbl[], w3892:dbl[], w3893:dbl[], w3906:dbl[], w3890:dbl[], w3904:dbl[], w3902:dbl[])
            n2035 = Negate(x=w3902) -> (-x=w3900:dbl[])
            n2036 = Divide(x=w3904, y=w3900) -> (x/y=w3903:dbl[])
            n2037 = Divide(x=w3893, y=w3890) -> (x/y=w3889:dbl[])
            n2038 = Divide(x=w3894, y=w3892) -> (x/y=w3891:dbl[])
            n2039 = Divide(x=w3941, y=w3939) -> (x/y=w3925:dbl[])
            n2040 = Divide(x=w3940, y=w3939) -> (x/y=w3924:dbl[])
            n2041 = Divide(x=w3938, y=w3936) -> (x/y=w3923:dbl[])
            n2042 = Divide(x=w3937, y=w3936) -> (x/y=w3922:dbl[])
            n2043 = Divide(x=w3908, y=w3892) -> (x/y=w3907:dbl[])
            n2044 = Divide(x=w3906, y=w3890) -> (x/y=w3905:dbl[])
            n2045 = Build Array(w3925, w3924, w3939, w3923, w3922, w3936, w3891, w3907, w3892, w3889, w3905, w3890, w3903, w3902) -> (w3901:dbl[][])
            n2046 = Bundle("T1 Y", "T1 X", "T1 Sum", "T2 Y", "T2 X", "T2 Sum", "T1 FB Y", "T1 FB X", "T1 FB Sum", "T2 FB Y", "T2 FB X", "T2 FB Sum", "PSD X", "PSD Y Sum") -> (w3888:T43)  [unwired: 1 out]
            n2047 = To Word Integer(number=w3943) -> (16bit integer=w3887:i16[])
            n2048 = Cluster To Array(cluster=w3888) -> (array=w3934:string[])
          }
        }
      }
    }
    "AI labels" <- w3020
    n2049 = Decimate 1D Array(w2994) -> (w3018:u32[], w2962:u32[])
    n2050 = local read "DMA Update Period (s)"() -> (w3030:dbl)
    n2051 = Build Array(w3018, w2962) -> (w3096:u32[][])
    n2052 = local read "Data Period (s)"() -> (w2868:dbl)
    n2053 = local read "BD 1 Frequency 2 (MHz)"() -> (w2901:dbl)
    n2054 = local read "BD 1 Frequency 1 (MHz)"() -> (w2902:dbl)
    n2055 = Decimate 1D Array(w2909) -> (w2933:i16[], w2932:i16[], w2930:i16[], w2929:i16[])  [unwired: 9 out]
    n2056 = To Double Precision Float(number=w3096) -> (double precision float=w3097:dbl[][])
    n2057 = local read "APD Integration Time (s)"() -> (w2975:dbl)
    n2058 = Multiply(x=w2868, y="Trap Pos. Disp. Downsample") -> (x*y=w2866:dbl)
    n2059 = Divide(x=w2933, y=w2932) -> (x/y=w2934:dbl[])
    n2060 = Divide(x=w2930, y=w2929) -> (x/y=w2931:dbl[])
    n2061 = feedback #6(0.0) -> (w2947:dbl)
    n2062 = Add(x=w3030, y=w2947) -> (x+y=w3136:dbl)
    n2063 = feedback-in #6(w3136) -> ()
    n2064 = local read "AOM X Cal (nm/MHz)"() -> (w2899:dbl)
    n2065 = To Time Stamp(1:w2947) -> (0:w2946:timestamp)
    n2066 = Split 1D Array(array=w2934, index="N El. to Ave.") -> (second subarray=w2937:dbl[])  [unwired: 1 out]
    n2067 = Split 1D Array(array=w2931, index="N El. to Ave.") -> (second subarray=w2936:dbl[])  [unwired: 1 out]
    n2068 = Multiply(x=w2868, y="Trap Disp. Downsample") -> (x*y=w2948:dbl)
    "Display Period (s)" <- w2948
    n2069 = for "Trap AI" {
      tunnel: [w3686] -> w3130 mode=indexing
      tunnel: w2946 -> [w3676]
      tunnel: "Trap Disp. Downsample" -> [w3684]
      tunnel: w3021 -> [w3682] mode=indexing
      tunnel: w2868 -> [w3681]
      tunnel: w3020 -> [w3680] mode=indexing
      tunnel: w2945 -> [w3679]
      tunnel: [w3678] -> w2986 mode=indexing
      tunnel: w2948 -> [w3677]
      workers-P: _ -> [_]
      n2070 = Bundle By Name("Y"=w3682, "dt"=w3681) -> (w3683:waveform(dbl))  [unwired: 1 out]
      n2071 = Set Waveform Attribute(5:w3680, 6:w3679, 7:w3683) -> (3:w3678:waveform(dbl))  [unwired: 1 in, 2 out]
      n2072 = call "downsample 1D array - double.vi"("Ave N"=w3684, "Array In"=w3682) -> ("Array Out"=w3685:dbl[])  [unwired: 1 out]
      n2073 = Bundle By Name(cluster=w3678, "t0"=w3676, "Y"=w3685, "dt"=w3677) -> (w3686:waveform(dbl))
    }
    n2074 = Bundle("BD 1 Frequency 1 (MHz)"=w2902, "BD 1 Frequency 2 (MHz)"=w2901) -> (w2903:T44)  [unwired: 1 out]
    n2075 = call <vilib>:"Mean.vi"("X"=w2936) -> ("mean"=w2924:dbl)  [unwired: 1 out]
    n2076 = call <vilib>:"Mean.vi"("X"=w2937) -> ("mean"=w2925:dbl)  [unwired: 1 out]
    n2077 = Reciprocal(x=w2948) -> (1/x=→"Trap Disp. Freq. (Hz)":dbl)
    n2078 = Cluster To Array(cluster=w2903) -> (array=w2900:dbl[])
    n2079 = local read "Trap X AI1 (DMA)"() -> (w2935:T13)
    n2080 = local read "Data points/scans (MCL)"() -> (w3108:dbl)
    n2081 = To Fixed-Point(number=w2924) -> (fixed-point=w2922:fxp<+/-,16,1>)  [unwired: 1 in]
    n2082 = To Fixed-Point(number=w2925) -> (fixed-point=w2923:fxp<+/-,16,1>)  [unwired: 1 in]
    n2083 = Bundle("Trap 1 Pos.", "Trap 2 Pos.") -> (w2944:cluster{string, string})  [unwired: 1 out]
    n2084 = Bundle By Name(cluster=w2935, "Set 1"=w2923, "Set 2"=w2922) -> (→"Trap X AI1 (DMA)":T13)
    n2085 = Cluster To Array(cluster=w2944) -> (array=w2941:string[])
    n2086 = Bundle("APD 1", "APD 2") -> (w3129:cluster{string, string})  [unwired: 1 out]
    n2087 = Select(t=-1.0, s="Negate Y Axis", f=1.0) -> (s? t:f=w2885:dbl)
    n2088 = for "Trap Position" {
      tunnel: w2950 -> [w3325] mode=indexing
      tunnel: "Trap Pos. Disp. Downsample" -> [w3324]
      tunnel: w2866 -> [w3322]
      tunnel: w2946 -> [w3321]
      tunnel: w2945 -> [w3319]
      tunnel: w2941 -> [w3318] mode=indexing
      tunnel: [w3317] -> w2855 mode=indexing
      tunnel: w2900 -> [w3315] mode=indexing
      tunnel: w2899 -> [w3313]
      tunnel: w2885 -> [w3312]
      n2089 = call "downsample 1D array - double.vi"("Ave N"=w3324, "Array In"=w3325) -> ("Array Out"=w3323:dbl[])  [unwired: 1 out]
      n2090 = Subtract(x=w3323, y=w3315) -> (x-y=w3316:dbl[])
      n2091 = Multiply(x=w3313, y=w3316) -> (x*y=w3314:dbl[])
      n2092 = Multiply(x=w3312, y=w3314) -> (x*y=w3311:dbl[])
      n2093 = Bundle By Name("Y"=w3311, "dt"=w3322, "t0"=w3321) -> (w3320:waveform(dbl))  [unwired: 1 out]
      n2094 = Set Waveform Attribute(5:w3318, 6:w3319, 7:w3320) -> (3:w3317:waveform(dbl))  [unwired: 1 in, 2 out]
    }
    n2095 = Cluster To Array(cluster=w3129) -> (array=w3126:string[])
    n2096 = for "APD" {
      tunnel: w3097 -> [w3665] mode=indexing
      tunnel: w2975 -> [w3673]
      tunnel: [w3669] -> w2982 mode=indexing
      tunnel: "APD Disp. Scale" -> [w3670]
      tunnel: w2945 -> [w3668]
      tunnel: w3126 -> [w3667] mode=indexing
      tunnel: "APD Disp. Downsample" -> [w3663]
      tunnel: [w3666] -> w3125
      workers-P: _ -> [_]
      tunnel: w2946 -> [w3662]
      n2097 = call "integrate 1D array interval - double.vi"("Ave N"=w3663, "Array In"=w3665) -> ("Array Out"=w3664:dbl[])  [unwired: 1 out]
      n2098 = Multiply(x=w3673, y=w3663) -> (x*y=w3666:dbl)
      n2099 = Divide(x=w3664, y=w3670) -> (x/y=w3671:dbl[])
      n2100 = Bundle By Name("t0"=w3662, "Y"=w3671, "dt"=w3666) -> (w3672:waveform(dbl))  [unwired: 1 out]
      n2101 = Set Waveform Attribute(5:w3667, 6:w3668, 7:w3672) -> (3:w3669:waveform(dbl))  [unwired: 1 in, 2 out]
    }
    "APD Display Period (s)" <- w3125
    n2102 = Reciprocal(x=w3125) -> (1/x=→"APD Display Freq. (Hz)":dbl)
    n2103 = local read "Display Period (s)"() -> (w3006:dbl)
    n2104 = Increment(x=w3108) -> (x+1=w3109:dbl)
    n2105 = To Double Precision Float(number=w3018) -> (double precision float=w3017:dbl[])
    n2106 = Index Array(array=w2855, index=0) -> (element=w2859:waveform(dbl))
    n2107 = Index Array(array=w2855, index=1) -> (element=w2854:waveform(dbl))
    n2108 = feedback #7(w3109) -> (w3112:dbl)
    n2109 = Select(t=0, s=w3099, f=w3112) -> (s? t:f=w3105:dbl)
    n2110 = Array Size(array=w3017) -> (size(s)=w3111:i32)
    n2111 = Add(x=w3111, y=w3105) -> (x+y=w3106:dbl)
    n2112 = Unbundle By Name(w2859) -> ("Y"=w2860:dbl[])
    n2113 = feedback #8(w3018) -> (w3095:u32[])
    n2114 = Build Array (concatenate)(w3095, w3018) -> (w3092:u32[])
    n2115 = feedback #9(w2962) -> (w2981:u32[])
    n2116 = Divide(x="Bead Sep. Int. Time (s)", y=w3006) -> (x/y=w2895:dbl)
    n2117 = Build Array (concatenate)(w2981, w2962) -> (w2980:u32[])
    n2118 = Add(x=w2860, y="FB Trap Pos Offset") -> (x+y=w2858:dbl[])
    "T1 x pos data" <- w2858
    n2119 = Greater?(x=w3106, y=w3108) -> (0:w3107:bool)
    n2120 = feedback #10(w2858) -> (w2897:dbl[])
    n2121 = Build Array (concatenate)(w2858, w2897) -> (w2896:dbl[])
    n2122 = Bundle By Name(cluster=w2859, "Y"=w2858) -> (w2857:waveform(dbl))
    n2123 = Select(t=w3105, s=w3107, f=w3106) -> (s? t:f=w3104:dbl)
    n2124 = feedback-in #7(w3104) -> ()
    n2125 = Array Size(array=w3092) -> (size(s)=w3089:i32)
    n2126 = Array Size(array=w3018) -> (size(s)=w3091:i32)
    n2127 = local read "MCL Scanning"() -> (w3102:bool)
    n2128 = local read "APD Integration Time (s)"() -> (w2989:dbl)
    n2129 = Bundle(w2857, w2854) -> (w2853:cluster{waveform(dbl), waveform(dbl)})  [unwired: 1 out]
    n2130 = Build Array (concatenate)(w2982, w3130) -> (w2984:waveform(dbl)[])
    "All Signals" <- w2984
    n2131 = Split 1D Array(array=w2896, index=w2895) -> (first subarray=w2889:dbl[])  [unwired: 1 out]
    n2132 = feedback-in #10(w2889) -> ()
    n2133 = Multiply(x=w3091, y="APD Ave N") -> (x*y=w3090:dbl)
    n2134 = Greater?(x=w3089, y=w3090) -> (0:w3093:bool)
    n2135 = Not(x=w3107) -> (.not. x?=w3101:bool)
    n2136 = Cluster To Array(cluster=w2853) -> (array=→"Trap Positions":waveform(dbl)[])
    n2137 = To Double Precision Float(number=w2962) -> (double precision float=w2961:dbl[])
    n2138 = call <vilib>:"Mean.vi"("X"=w2889) -> ("mean"=w2888:dbl)  [unwired: 1 out]
    "Mean T1 Position (nm)" <- w2888
    n2139 = Subtract(x=w2889, y=w2888) -> (x-y=w2894:dbl[])
    n2140 = Square(x=w2894) -> (x^2=w2893:dbl[])
    n2141 = And(x=w3101, y=w3102) -> (x .and. y?=w3103:bool)
    n2142 = call <vilib>:"Mean.vi"("X"=w2893) -> ("mean"=w2892:dbl)  [unwired: 1 out]
    n2143 = case shown="True" w3093 {
      tunnel: w3092 -> [w3445 w3452]
      tunnel: [w3445 w3450] -> w3035
      tunnel: w3090 -> [_ w3447]
      tunnel: w3089 -> [_ w3451]
      tunnel: w2980 -> [w3444 w3449]
      tunnel: [w3444 w3446] -> w2977
      frame False {
      }
      frame True {
        n2144 = Subtract(x=w3451, y=w3447) -> (x-y=w3448:dbl)
        n2145 = Array Subset(array=w3452, index=w3448, length=w3447) -> (w3450:u32[])
        n2146 = Array Subset(array=w3449, index=w3448, length=w3447) -> (w3446:u32[])
      }
    }
    n2147 = feedback-in #8(w3035) -> ()
    n2148 = feedback-in #9(w2977) -> ()
    n2149 = Square Root(x=w2892) -> (sqrt(x)=w2891:dbl)
    n2150 = Or(x=w3103, y=w3099) -> (x .or. y?=w3100:bool)
    n2151 = Equal?(x="Tab Control 6", y=T34."High Res Display") -> (x = y?=w3024:bool)
    n2152 = Multiply(x="APD Disp. Scale", y=w2982) -> (x*y=w2991:waveform(dbl)[])
    n2153 = Multiply(x=10.0, y=w2891) -> (x*y=→"Trap 1 Position RMS (A)":dbl)
    n2154 = Multiply(x="APD Disp. Downsample", y=w2989) -> (x*y=w2987:dbl)
    n2155 = Divide(x=w2991, y=w2987) -> (x/y=w2959:waveform(dbl)[])
    n2156 = case "For displaying the high resolution display (no downsampling)" shown="True" w3024 {
      tunnel: w2986 -> [_ w3345]
      frame False {
      }
      frame True {
        n2157 = Index Array(array=w3345, index="High Res. Display") -> (element=w3346:waveform(dbl))
        n2158 = call <vilib>:"Std Deviation and Variance.vi"("X"=w3346) -> ("mean"=w3353:dbl, "standard deviation"=w3358:dbl)  [unwired: 1 in, 1 out]
        "Mean Intensity" <- w3353
        "Sigma" <- w3358
        n2159 = Subtract(x=w3346, y=w3353) -> (x-y=w3352:waveform(dbl))
        n2160 = Select(t=w3352, s="Subtract mean", f=w3346) -> (s? t:f=→"1 Channel":waveform(dbl))
        n2161 = Divide(x=w3358, y=w3353) -> (x/y=→"Sigma/Mean":dbl)
        n2162 = feedback #11(1) -> (w3347:i32)
        n2163 = Greater Or Equal?(x=w3347, y="Slow mean N ave.") -> (x >= y?=w3360:bool)
        n2164 = Increment(x=w3347) -> (x+1=w3362:i32)
        n2165 = Select(t=1, s=w3360, f=w3362) -> (s? t:f=w3349:i32)
        n2166 = feedback-in #11(w3349) -> ()
        n2167 = feedback #12() -> (w3350:waveform(dbl))  [unwired: 1 out]
        n2168 = case shown="Default" w3347 {
          tunnel: [w3365 w3368] -> w3351
          tunnel: w3350 -> [w3367 _]
          tunnel: w3346 -> [w3366 w3368]
          frame Default {
            n2169 = call-poly <vilib>:"Append Waveforms.vi"("waveform B"=w3366, "waveform A"=w3367) -> ("waveform out"=w3365:waveform(dbl))  [unwired: 1 in, 8 out]
          }
          frame 1 {
          }
        }
        n2170 = feedback-in #12(w3351) -> ()
        n2171 = case shown="True" w3360 {
          tunnel: w3351 -> [_ w3364]
          frame False {
          }
          frame True {
            n2172 = call <vilib>:"Mean.vi"("X"=w3364) -> ("mean"=→"Slow mean":dbl)  [unwired: 1 out]
          }
        }
      }
    }
    n2173 = Index Array(array=w2959, index=0) -> (element=w2969:waveform(dbl))
    n2174 = Index Array(array=w2959, index=1) -> (element=w2967:waveform(dbl))
    n2175 = case "For computing FFTs for display" shown="True" "Compute FFT" {
      tunnel: w2986 -> [_ w4059]
      frame False {
      }
      frame True {
        n2176 = Build Array("FFT 1 Choice 1", "FFT 1 Choice 2", "FFT 2 Choice 1", "FFT 2 Choice 2") -> (w4052:u16[])
        n2177 = Array Size(array=w4059) -> (size(s)=w4058:i32)
        n2178 = feedback-in #13(w4052) -> ()
        n2179 = feedback #13(u16[] [100, 100, 100, 100]) -> (w4053:u16[])
        n2180 = feedback-in #14("# Spectra to Ave.") -> ()
        n2181 = feedback #14("# Spectra to Ave.") -> (w4050:dbl)
        n2182 = Not Equal?(x="# Spectra to Ave.", y=w4050) -> (x != y?=w4049:bool)
        n2183 = Not Equal?(x=w4052, y=w4053) -> (x != y?=w4051:bool)
        n2184 = feedback #15(1.0) -> (w4036:dbl)
        n2185 = Compound Arithmetic op=OR("Reset FFT", w4051, w4049) -> (w4034:bool)
        n2186 = Select(t=1.0, s=w4034, f=w4036) -> (s? t:f=w4038:dbl)
        n2187 = Greater?(x=w4038, y="# Spectra to Ave.") -> (0:w4057:bool)
        n2188 = Increment(x=w4038) -> (x+1=w4037:dbl)
        n2189 = feedback-in #15(w4037) -> ()
        n2190 = local read "DMA Update Period (s)"() -> (w4032:dbl)
        n2191 = Multiply(x="# Spectra to Ave.", y=w4032) -> (x*y=→"Ave. Time (s)":dbl)
        n2192 = Build Array(cluster{"f0":dbl, "df":dbl, "magnitude":dbl[]} {"f0"=0.0, "df"=0.0, "magnitude"=[]} ("PSD")) -> (w4041:cluster{"f0":dbl, "df":dbl, "magnitude":dbl[]}[])
        n2193 = Build Array(w4041, w4041, w4041, w4041) -> (w4043:T45)
        n2194 = feedback #16(w4043) -> (w4048:T45)
        n2195 = for {
          N: 4 -> [_]
          tunnel: w4052 -> [w4081] mode=indexing
          tunnel: w4059 -> [w4082]
          tunnel: w4058 -> [w4084]
          tunnel: w4034 -> [w4077]
          tunnel: w4057 -> [w4076]
          tunnel: "# Spectra to Ave." -> [w4075]
          tunnel: [w4074] -> w4047 mode=indexing
          tunnel: w4048 -> [w4079] mode=indexing
          tunnel: [w4078] -> w4035 mode=indexing
          tunnel: w4038 -> [w4073]
          n2196 = Less?(x=w4081, y=w4084) -> (x < y?=w4083:bool)
          n2197 = Index Array(array=w4082, index=w4081) -> (element=w4080:waveform(dbl))
          n2198 = case shown="True" w4083 {
            tunnel: w4080 -> [_ w4101]
            tunnel: w4079 -> [w4086 w4099]
            tunnel: [w4086 w4087] -> w4078
            tunnel: w4077 -> [_ w4098]
            tunnel: w4076 -> [_ w4091]
            tunnel: w4075 -> [_ w4090]
            tunnel: [cluster{"f0":dbl, "df":dbl, "magnitude":dbl[]} {"f0"=0.0, "df"=0.0, "magnitude"=[]} ("PSD") w4092] -> w4074
            tunnel: w4073 -> [_ w4089]
            frame False {
            }
            frame True {
              n2199 = call <vilib>:"Std Deviation and Variance.vi"("X"=w4101) -> ("mean"=w4102:dbl)  [unwired: 1 in, 2 out]
              n2200 = Subtract(x=w4101, y=w4102) -> (x-y=w4100:waveform(dbl))
              n2201 = xnode "Spectral Measurements"("Signals"=w4100) -> ("PSD"=w4094:cluster{"f0":dbl, "df":dbl, "magnitude":dbl[]})  [unwired: 1 in, 1 out]
              n2202 = case shown="False" w4098 {
                tunnel: w4099 -> [w4111 _]
                tunnel: [w4107 w4116] -> w4087
                tunnel: w4094 -> [w4110 w4117]
                tunnel: w4091 -> [w4109 _]
                frame False {
                  n2203 = Build Array (concatenate)(w4111, w4110) -> (w4108:cluster{"f0":dbl, "df":dbl, "magnitude":dbl[]}[])
                  n2204 = case shown="True" w4109 {
                    tunnel: w4108 -> [w4112 w4115]
                    tunnel: [w4112 w4113] -> w4107
                    frame False {
                    }
                    frame True {
                      n2205 = Delete From Array(array=w4115, index=0) -> (array with subset deleted=w4113:cluster{"f0":dbl, "df":dbl, "magnitude":dbl[]}[])  [unwired: 1 in, 1 out]
                    }
                  }
                }
                frame True {
                  n2206 = Build Array(w4117) -> (w4116:cluster{"f0":dbl, "df":dbl, "magnitude":dbl[]}[])
                }
              }
              n2207 = for {
                tunnel: w4087 -> [w4106] mode=indexing
                tunnel: [w4105] -> w4097 mode=indexing
                workers-P: _ -> [_]
                n2208 = Unbundle By Name(w4106) -> ("magnitude"=w4105:dbl[])
              }
              n2209 = Transpose 2D Array(2D array=w4097) -> (transposed array=w4096:dbl[][])
              n2210 = for {
                tunnel: w4096 -> [w4104] mode=indexing
                tunnel: [w4103] -> w4095 mode=indexing
                workers-P: _ -> [_]
                n2211 = Add Array Elements(numeric array=w4104) -> (sum=w4103:dbl)
              }
              n2212 = Select(t=w4090, s=w4091, f=w4089) -> (s? t:f=w4088:dbl)
              n2213 = Divide(x=w4095, y=w4088) -> (x/y=w4093:dbl[])
              n2214 = Bundle By Name(cluster=w4094, "magnitude"=w4093) -> (w4092:cluster{"f0":dbl, "df":dbl, "magnitude":dbl[]})
            }
          }
        }
        n2215 = case shown="True" w4034 {
          tunnel: w4035 -> [w4066 w4072]
          tunnel: [w4066 w4067] -> w4033
          frame False {
          }
          frame True {
            n2216 = Array Subset(array=w4072, index (row)=0 ("index"), length (row)=4 ("length"), index (col)=0 ("index"), length (col)=1 ("length")) -> (w4067:T45)
          }
        }
        n2217 = feedback-in #16(w4033) -> ()
        n2218 = Split 1D Array(array=w4047, index=2) -> (first subarray=→"FFT 1":cluster{"f0":dbl, "df":dbl, "magnitude":dbl[]}[], second subarray=→"FFT 2":cluster{"f0":dbl, "df":dbl, "magnitude":dbl[]}[])
      }
    }
    n2219 = case "For plotting results of scanning MCL" shown="True" w3100 {
      tunnel: w3099 -> [_ w3485]
      tunnel: w3017 -> [_ w3581]
      tunnel: w3108 -> [_ _]
      tunnel: w2986 -> [_ w3555]
      tunnel: w2961 -> [_ w3486]
      tunnel: w2960 -> [_ w3459]
      frame False {
      }
      frame True {
        w3466 = u32 0 items=["Horizontal", "Vertical", "Central", "1st Diagonal", "2nd Diagonal"] ("Type of Symmetry")
        w3494 = u32 0 items=["Horizontal", "Vertical", "Central", "1st Diagonal", "2nd Diagonal"] ("Type of Symmetry")
        w3497 = u32 0 items=["Horizontal", "Vertical", "Central", "1st Diagonal", "2nd Diagonal"] ("Type of Symmetry")
        w3526 = u32 0 items=["Horizontal", "Vertical", "Central", "1st Diagonal", "2nd Diagonal"] ("Type of Symmetry")
        n2220 = Index Array(array=w3555, index=10) -> (element=w3561:waveform(dbl))
        n2221 = Index Array(array=w3555, index=11) -> (element=w3558:waveform(dbl))
        n2222 = local read "Cycles/step (MCL)"() -> (w3511:u64)
        n2223 = Index Array(array=w3555, index="Channel") -> (element=w3557:waveform(dbl))
        n2224 = Unbundle(w3459) -> ("New Image"=w3458:T2, "New Image"=w3457:T2, "New Image"=w3456:T2, "New Image"=w3455:T2)
        n2225 = Unbundle By Name(w3561) -> ("Y"=w3513:dbl[])
        n2226 = Unbundle By Name(w3558) -> ("Y"=w3515:dbl[])
        n2227 = Unbundle By Name(w3557) -> ("Y"=w3520:dbl[])
        n2228 = call "downsample 1D array - double.vi"("Ave N"=w3511, "Array In"=w3513) -> ("Array Out"=w3512:dbl[])  [unwired: 1 out]
        n2229 = call "downsample 1D array - double.vi"("Ave N"=w3511, "Array In"=w3515) -> ("Array Out"=w3514:dbl[])  [unwired: 1 out]
        n2230 = call "downsample 1D array - double.vi"("Ave N"=w3511, "Array In"=w3520) -> ("Array Out"=w3519:dbl[])  [unwired: 1 out]
        n2231 = feedback #17(w3581) -> (w3582:dbl[])
        n2232 = Build Array (concatenate)(w3582, w3581) -> (w3563:dbl[])
        n2233 = feedback #18(w3486) -> (w3488:dbl[])
